vi "TempRamp.vi"() -> ()   [LabVIEW 2016]
uses:
  <vilib>/addons/control/pid/pid.llb/PID (DBL).vi
  <vilib>/addons/control/pid/NI_PID_pid.lvlib
panel:
  out "Power Supply Output":dbl
  out "Thermocouple (mV) 2":dbl
  in  "Max .Temp. (mV)":dbl
  in  "Max. Power Output (0-10)":dbl
  in  "PID parameters":T1={"proportional gain (Kc)"=1.0, "integral time (Ti, min)"=0.01, "derivative time (Td, min)"=0.0} {"derivative time (Td, min)" format="%.3f"; "integral time (Ti, min)" format="%.3f"; "proportional gain (Kc)" format="%.3f"}
  in  "Safety Button":bool
  in  "Initial Temp. (mV)":dbl
  in  "Slope (mV/s)":dbl
  out "Time bar":u8(slide) scale=0.0..100.0
  out "Elapsed Time":dbl caption="Elapsed Time (s)"
  in  "Duration (s)":dbl=60.0 caption="Time Target (s)"
  out "XY Graph":cluster{"Y":dbl[], "Y":dbl[]}[](graph)
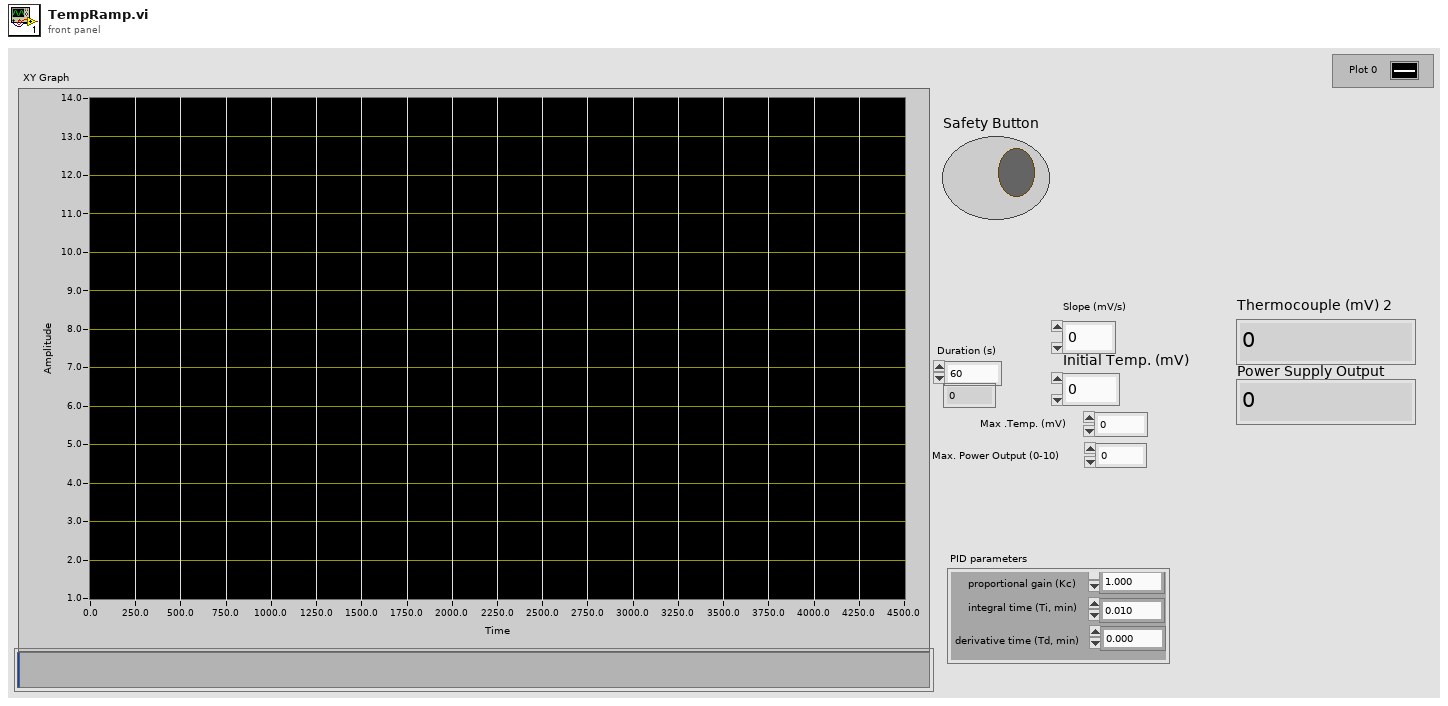
[diagram p1: front panel]
types:
  T1 = cluster{"proportional gain (Kc)":dbl, "integral time (Ti, min)":dbl, "derivative time (Td, min)":dbl}
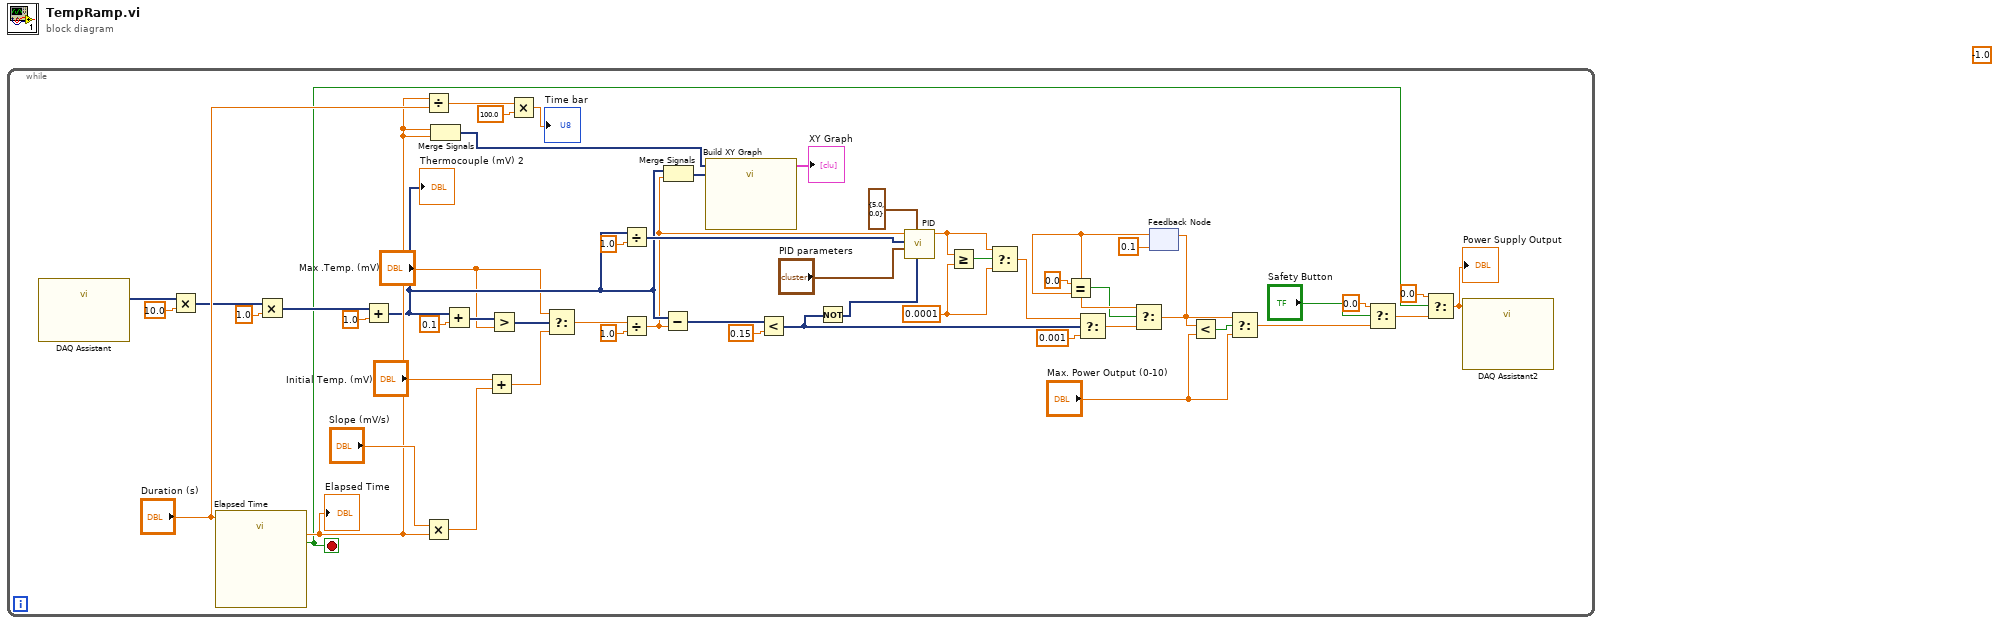
[diagram p0: block diagram]
diagram:
  (unwired) -1.0
  n1 = while {
    stop <- w10 stop-if-true
    w42 = 0.0001 ("Minimum Power Supply Factor")
    n2 = call "DAQ Assistant"() -> ("data"=w31:dynamicdata)  [unwired: 17 in, 2 out]
    n3 = Multiply(x=w31, y=10.0) -> (x*y=w40:dynamicdata)
    n4 = call "Elapsed Time"("Time Target (s)"="Duration (s)") -> ("Elapsed Time (s)"=w11:dbl, "Time has Elapsed"=w10:bool)  [unwired: 11 in, 6 out]
    "Elapsed Time" <- w11
    n5 = Multiply(x=w40, y=1.0) -> (x*y=w44:dynamicdata)
    n6 = Add(x=w44, y=1.0) -> (x+y=w7:dynamicdata)
    "Thermocouple (mV) 2" <- w7
    n7 = Divide(x=w11, y="Duration (s)") -> (x/y=w54:dbl)
    n8 = Multiply(x="Slope (mV/s)", y=w11) -> (x*y=w50:dbl)
    n9 = Merge Signals(w11, w11) -> (w12:dynamicdata)
    n10 = Add(x=w7, y=0.1) -> (x+y=w4:dynamicdata)
    n11 = Add(x="Initial Temp. (mV)", y=w50) -> (x+y=w6:dbl)
    n12 = Greater?(x=w4, y="Max .Temp. (mV)") -> (0:w9:dynamicdata)
    n13 = Multiply(x=w54, y=100.0) -> (x*y=→"Time bar":dbl)
    n14 = Select(t="Max .Temp. (mV)", s=w9, f=w6) -> (s? t:f=w5:dbl)
    n15 = Divide(x=w7, y=1.0) -> (x/y=w17:dynamicdata)
    n16 = Divide(x=w5, y=1.0) -> (x/y=w3:dbl)
    n17 = Subtract(x=w7, y=w3) -> (x-y=w38:dynamicdata)
    n18 = Merge Signals(w7, w3) -> (w13:dynamicdata)
    n19 = call "Build XY Graph"("Y Input"=w13, "X Input"=w12) -> ("XY Graph"=→"XY Graph":cluster{"Y":dbl[], "Y":dbl[]}[])  [unwired: 3 in, 6 out]
    n20 = Less?(x=w38, y=0.15) -> (x < y?=w16:dynamicdata)
    n21 = Not(x=w16) -> (.not. x?=w15:dynamicdata)
    n22 = call-poly <vilib>:"PID.vi"("reinitialize? (F)"=w15, "output range"=cluster{"output high":dbl, "output low":dbl} {"output high"=5.0, "output low"=0.0}, "PID gains"="PID parameters", "process variable"=w17, "setpoint"=w3) -> ("output"=w22:dbl)  [unwired: 5 in, 1 out]
    n23 = Greater Or Equal?(x=w22, y=w42) -> (x >= y?=w46:bool)
    n24 = Select(t=w22, s=w46, f=w42) -> (s? t:f=w8:dbl)
    n25 = Select(t=w8, s=w16, f=0.001) -> (s? t:f=w25:dbl)
    n26 = feedback #1(0.1 ("f")) -> (w27:dbl)
    n27 = Equal?(x=0.0, y=w27) -> (x = y?=w26:bool)
    n28 = Select(t=w27, s=w26, f=w25) -> (s? t:f=w24:dbl)
    n29 = feedback-in #1(w24) -> ()
    n30 = Less?(x=w24, y="Max. Power Output (0-10)") -> (x < y?=w35:bool)
    n31 = Select(t=w24, s=w35, f="Max. Power Output (0-10)") -> (s? t:f=w34:dbl)
    n32 = Select(t=0.0, s="Safety Button", f=w34) -> (s? t:f=w33:dbl)
    n33 = Select(t=0.0, s=w10, f=w33) -> (s? t:f=w47:dbl)
    "Power Supply Output" <- w47
    n34 = call "DAQ Assistant2"("data"=w47) -> ()  [unwired: 17 in, 2 out]
  }
